vi "Images.vi"() -> ()   [LabVIEW 2015]
panel:
  in  "Image 3":T1(plugin-control)=refnum
  in  "Image":T1(plugin-control)=refnum
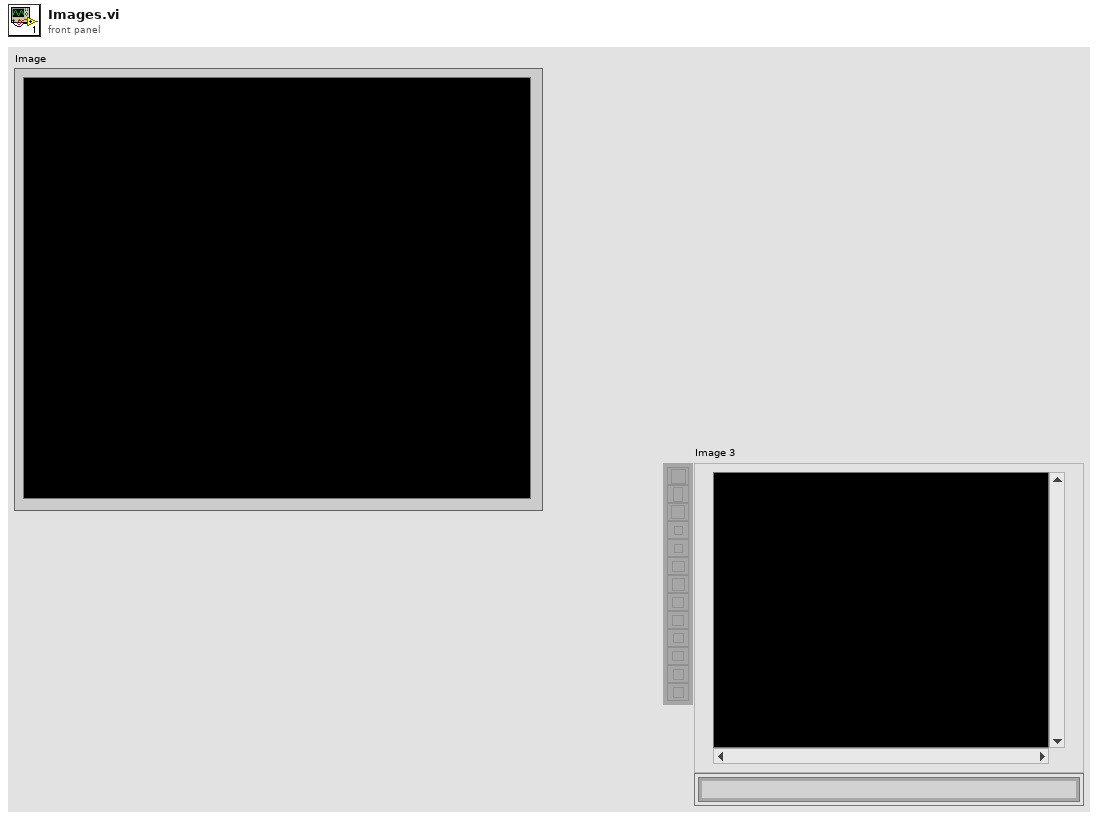
[diagram p1: front panel]
types:
  T1 = typedef "IMAQ Image.ctl" = refnum<image>
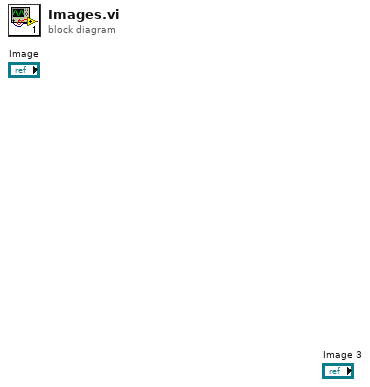
[diagram p0: block diagram]
diagram:
